vi "Toggle on Release.vi"(11 "Boolean":bool) -> (3 "toggle on release":bool)   [LabVIEW 2018]
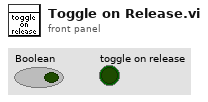
[diagram p1: front panel]
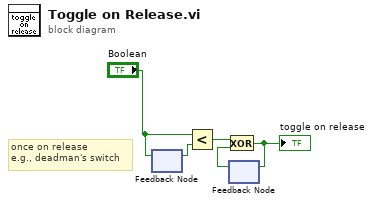
[diagram p0: block diagram]
diagram:
  # "once on release\ne.g., deadman's switch"
  n1 = feedback #1() -> (w4:bool)  [unwired: 1 in]
  n2 = feedback-in #1("Boolean") -> ()
  n3 = Less?(x="Boolean", y=w4) -> (x < y?=w2:bool)
  n4 = feedback #2() -> (w1:bool)  [unwired: 1 in]
  n5 = Exclusive Or(1:w1, 2:w2) -> (0:w3:bool)
  "toggle on release" <- w3
  n6 = feedback-in #2(w3) -> ()
